vi "PLL Freq Modulation.vi"(8 "norminal freq [U16.0]":fxp<+,16,0>, 9 "reset?":bool, 10 "alpha [U16.0]":fxp<+,16,0>, 11 "x[I16.2(changed)]":fxp<+/-,16,2>) -> (0 "f":fxp<+/-,32,0> format="%.32g", 1 "z [I32.1]":fxp<+/-,32,1>, 2 "sin(z)":fxp<+/-,16,2> format="%.15g", 3 "cos(z)":fxp<+/-,16,2> format="%.15g")   [LabVIEW 2012]
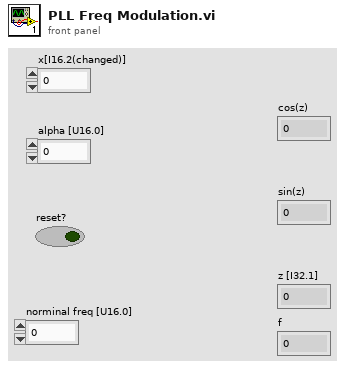
[diagram p1: front panel]
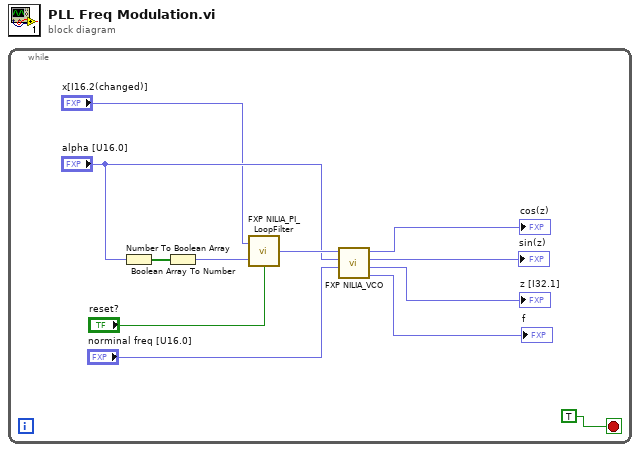
[diagram p0: block diagram]
diagram:
  n1 = while {
    stop <- TRUE stop-if-true
    n2 = Number To Boolean Array(number="alpha [U16.0]") -> (Boolean array=w9:bool[])
    n3 = Boolean Array To Number(Boolean array=w9) -> (number=w8:fxp<+,16,-2>)
    n4 = call "FXP NILIA_PI_LoopFilter.vi"("reset?"="reset?", "alpha [U16.-2]"=w8, "x [I16.2]"="x[I16.2(changed)]") -> ("x+y [I32.17]"=w12:fxp<+/-,32,17>)
    n5 = call "FXP NILIA_VCO.vi"("nominal freq [U16.0]"="norminal freq [U16.0]", "Kv [U16.0]"="alpha [U16.0]", "v [I32.17]"=w12) -> ("f"=→"f":fxp<+/-,32,0>, "z [I32.1]"=→"z [I32.1]":fxp<+/-,32,1>, "sin(z) [I16.2]"=→"sin(z)":fxp<+/-,16,2>, "cos(z) [I16.2]"=→"cos(z)":fxp<+/-,16,2>)  [unwired: 5 out]
  }
